vi "GetFill.vi"(8 "error in (no error)":errorcluster, 11 "Circle in":refnum<class "Circle.lvclass">) -> (0 "error out":errorcluster, 2 "Fill":bool, 3 "Circle out":refnum<class "Circle.lvclass">)   [LabVIEW 2021, in "Picture2D.lvlib" / "Circle.lvclass"]
uses:
  Circle.lvclass
  Circle.lvclass/Circle.ctl
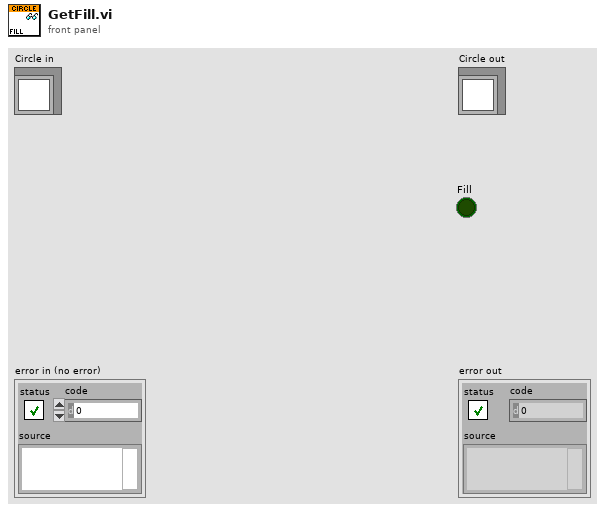
[diagram p1: front panel]
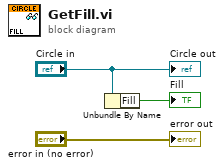
[diagram p0: block diagram]
diagram:
  n1 = Unbundle By Name("Circle in") -> ("Fill"=→"Fill":bool)
  "error out" <- "error in (no error)"
  "Circle out" <- "Circle in"
